vi "0xEA_Cmd_read_one_float_parameter_(SubVI).vi"(10 "Номер считываемого параметра float":i32, 11 "String in":string) -> (3 "String out":string)   [LabVIEW 2017, in "LV_Unicorn.lvlib"]
uses:
  LV_Unicorn.lvlib
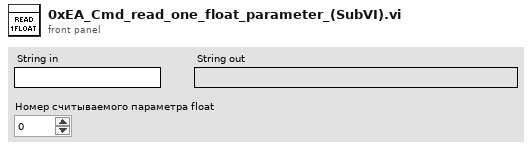
[diagram p1: front panel]
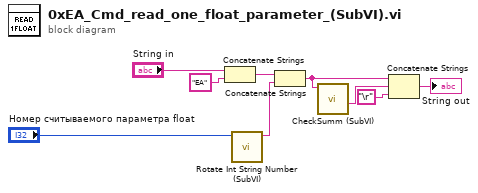
[diagram p0: block diagram]
diagram:
  n1 = Concatenate Strings("String in", "EA" ("string")) -> (w7:string)
  n2 = call "Rotate Int String Number (SubVI).vi"("Int Number In"="Номер считываемого параметра float") -> ("Orig String"=w2:string)  [unwired: 8 in, 2 out]
  n3 = Concatenate Strings(w7, w2) -> (w4:string)
  n4 = call "CheckSumm (SubVI).vi"("Input String"=w4) -> ("CheckSumm"=w3:string)  [unwired: 7 in, 3 out]
  n5 = Concatenate Strings(w4, w3, "\r") -> (→"String out":string)
